vi "GluePattern_Positioning(SubVI)_old.vi"(4 "Duration of glue \ndispensing [s]":dbl=1.5, 5 "File to be processed- Dots":path=path "C:/Users/Aerotech/Documents/BNL_ThermomechanicalStave/1_ModulePlacement/1_GluePatterning/LabVIEW_gluepattern_arraytest.csv", 6 "Type of Pattern":u16(ring) items=["Dots", "Lines"], 7 "Go to \ncoordinates":T5={"X [mm]"=10.0, "Y [mm]"=-17.0, "Z [mm] "=36.0}) -> ()   [LabVIEW 2016]
uses:
  C:/Users/Aerotech/Documents/BNL_ThermomechanicalStave/AerotechLibraries/Bin/Aerotech.A3200.dll
  AerotechLibraries/Bin/Aerotech.A3200.dll
  <vilib>/LabVIEW Interface for Arduino/Type Defs/Arduino Resource.ctl
  <vilib>/LabVIEW Interface for Arduino/Type Defs/Board Type.ctl
  <vilib>/LabVIEW Interface for Arduino/Type Defs/Pin Mode.ctl
  <vilib>/Utility/file.llb/Read Delimited Spreadsheet (DBL).vi
  <vilib>/LabVIEW Interface for Arduino/LabVIEW Interface for Arduino.lvlib
panel:
  out "error out":errorcluster
  out "DX [mm]":dbl
  out "DY [mm]":dbl
  out "Arduino Resource":T1={"VISA resource"="COM3", "Board Type"=enum."Uno", "Connection Type"=enum."USB / Serial", "Bytes Per Packet (15)"=15}
  in  "Digital I/O Pin":u8=7
  in  "Final Z":dbl=41.0
  out "Final Position":T3={"Final X"=10.000061631047261, "Final Y"=-16.999877872052817, "Final Z"=35.999801000000005}
  out "Column":i32
  out "Row":i32
  in  "Home?":bool
  out "XYZ Stage Control":refnum<k24>
  in  "Axis Speeds":T4={"vX [mm]"=40.0, "vY [mm]"=40.0, "vZ [mm] "=40.0}
  in  "Module width [mm]":dbl
  in  "Module length [mm]":dbl
  out "INPUT : Dot":bool[][](array[boolean])=[[TRUE]]
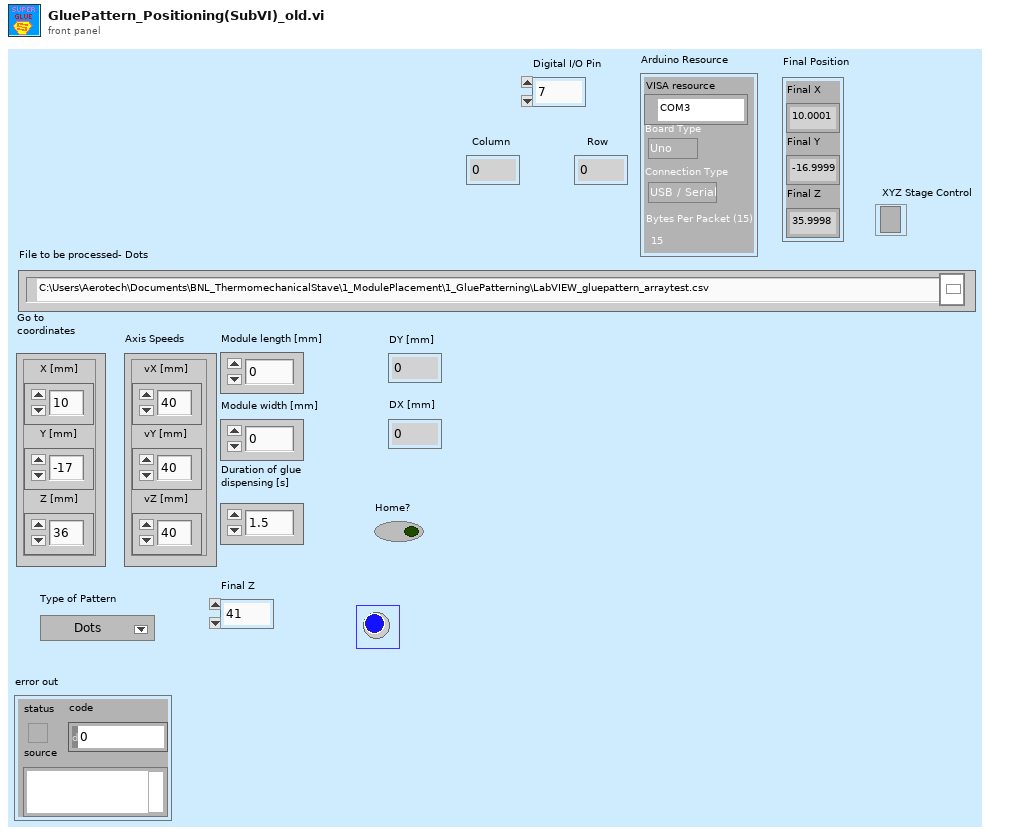
[diagram p1: front panel]
types:
  T1 = typedef "LabVIEW Interface for Arduino.lvlib/Arduino Resource.ctl" = cluster{"VISA resource":refnum<visa-resource-name>, "Board Type":T2, "Connection Type":enum8{"USB / Serial"}, "Bytes Per Packet (15)":u8}
  T2 = typedef "LabVIEW Interface for Arduino.lvlib/Board Type.ctl" = enum16{"Uno", "Dimuelanove w/Atmega 328", "Mega 2560"}
  T3 = cluster{"Final X":dbl, "Final Y":dbl, "Final Z":dbl}
  T4 = cluster{"vX [mm]":dbl, "vY [mm]":dbl, "vZ [mm] ":dbl}
  T5 = cluster{"X [mm]":dbl, "Y [mm]":dbl, "Z [mm] ":dbl}
  T6 = typedef "LabVIEW Interface for Arduino.lvlib/Pin Mode.ctl" = enum8{"Input", "Output"}
  T7 = cluster{"X [mm]":dbl, "Y [mm]":dbl, "Z [mm]":dbl}
  T8 = cluster{"X Position Feedback":dbl, "Y Position Feedback":dbl, "Z Position Feedback":dbl}
  T9 = cluster{"Final X":dbl, "Final Y":dbl, "Z [mm] ":dbl}
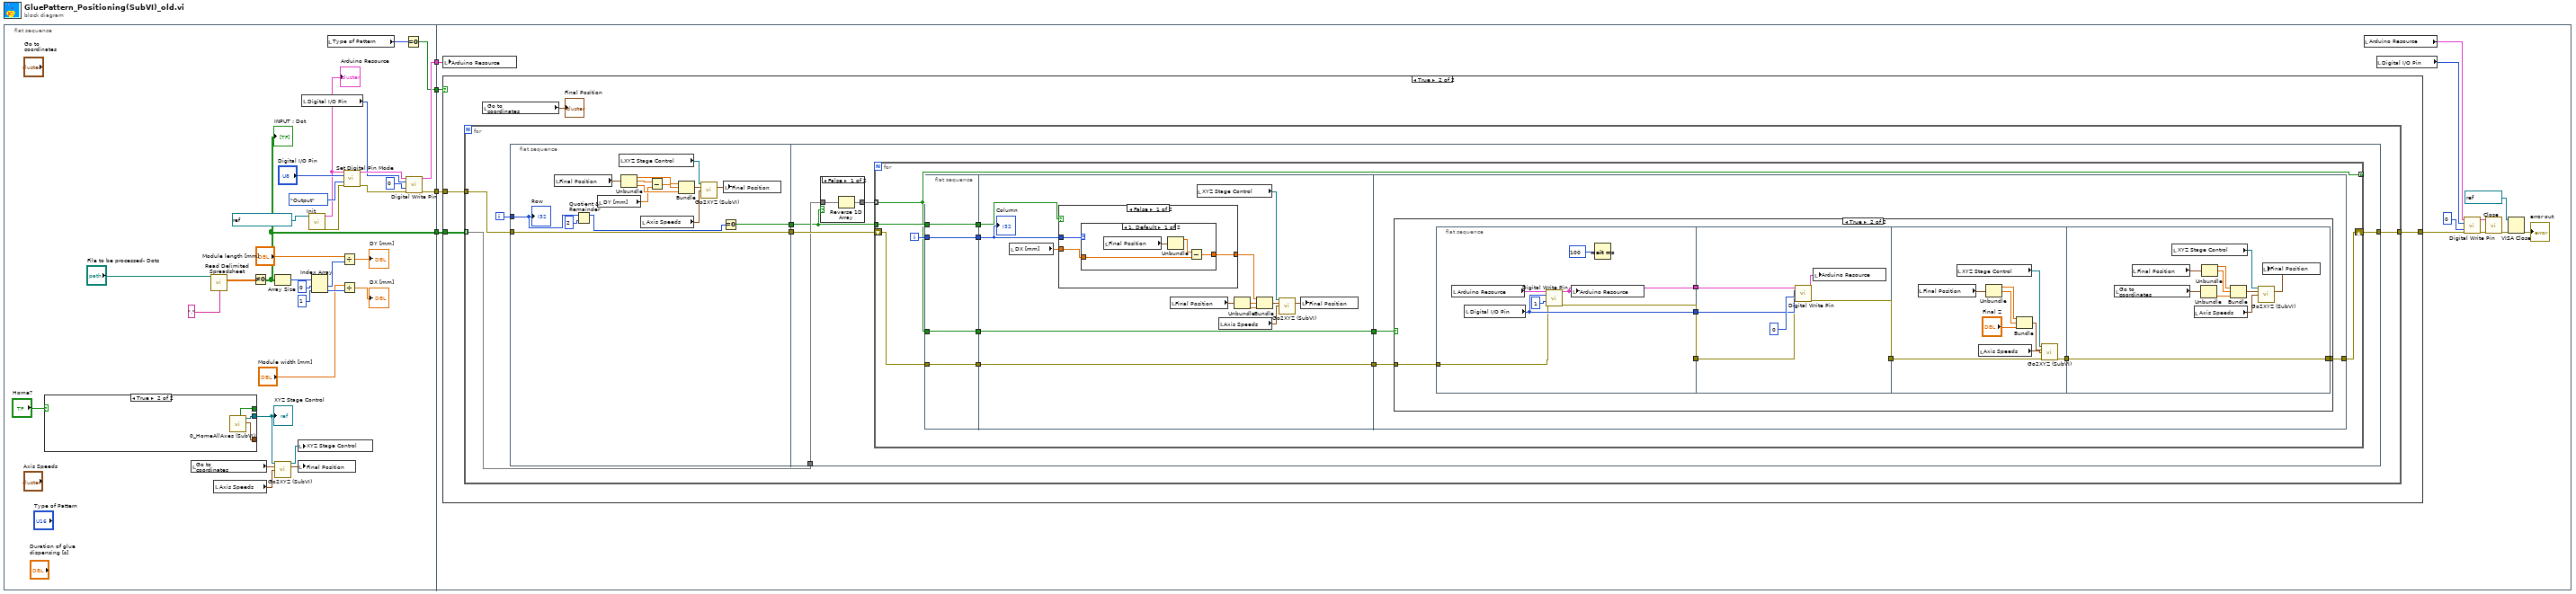
[diagram p0: block diagram]
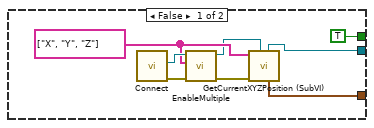
[diagram p2: hidden frame]
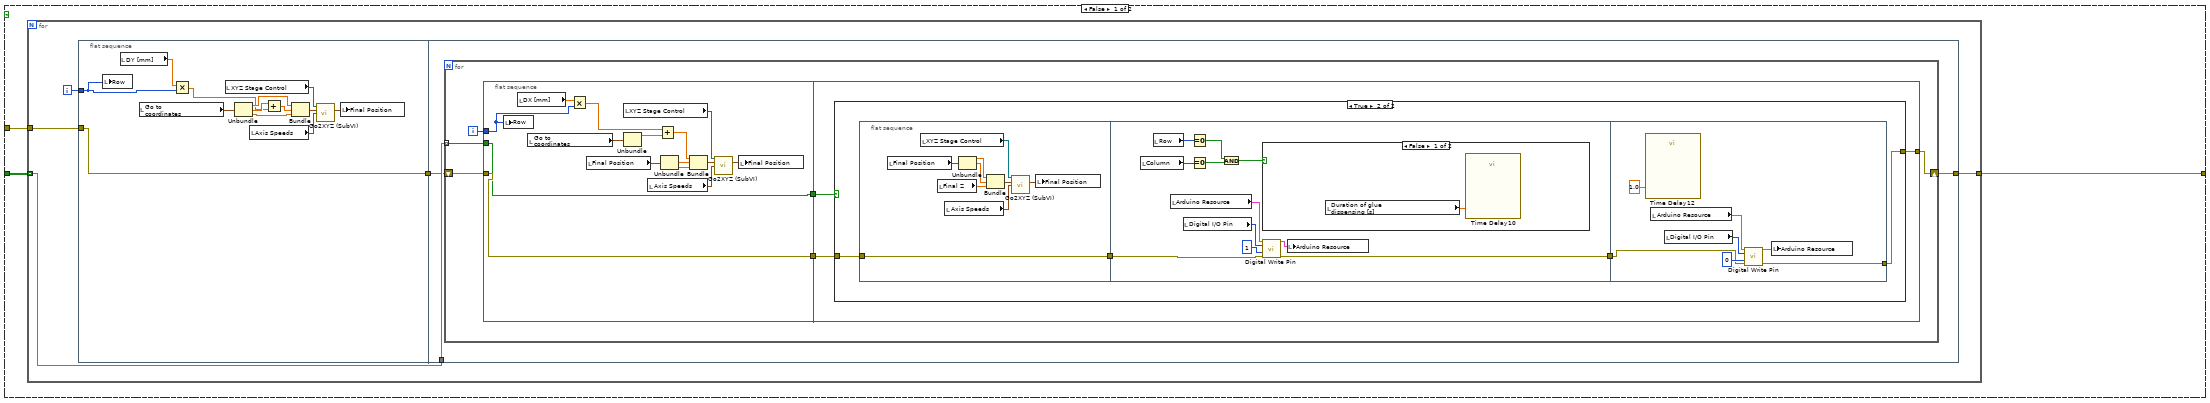
[diagram p3: hidden frame]
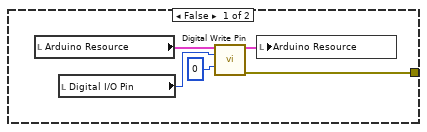
[diagram p4: hidden frame]
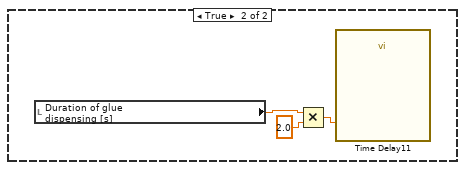
[diagram p5: hidden frame]
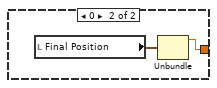
[diagram p7: hidden frame]
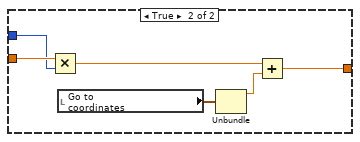
[diagram p8: hidden frame]
diagram:
  n1 = flat-sequence {
    tunnel: [w36] -> w4
    tunnel: [w10] -> w3
    tunnel: [w5] -> w2
    tunnel: [w7] -> w1
    tunnel: w4 -> [w60]
    tunnel: w3 -> [w58]
    tunnel: w2 -> [w59]
    tunnel: w1 -> [w57]
    frame #0 {
      n2 = case shown="True" "Home?" {
        tunnel: [w37 w47] -> _
        tunnel: [TRUE ("completed") w46] -> _
        tunnel: [w39 w45] -> w23
        frame False {
          w41 = string[] ["X", "Y", "Z"] ("Axes Names")
          n3 = call "Connect.vi"() -> ("error out"=w43:errorcluster, "controller"=w42:refnum<k24>)  [unwired: 10 in]
          n4 = call "EnableMultiple.vi"("error in (no error)"=w43, "axis names"=w41, "controller in"=w42) -> ("error out"=w44:errorcluster, "controller out"=w40:refnum<k24>)  [unwired: 7 in]
          n5 = call "GetCurrentXYZPosition (SubVI).vi"(".NET Refnum in - Device"=w40, "error in (no error)"=w44, "Axes Names"=w41) -> ("Current stage position"=w37:T7, ".NET Refnum out  - Device"=w39:refnum<k24>)  [unwired: 3 in, 4 out]
        }
        frame True {
          n6 = call "0_HomeAllAxes (SubVI).vi"() -> ("Homed coordinates"=w47:T8, "controller out"=w45:refnum<k24>, "completed"=w46:bool)  [unwired: 8 in, 1 out]
        }
      }
      "XYZ Stage Control" <- w23
      n7 = local read "Go to \ncoordinates"() -> (w18:T5)
      n8 = call-poly <vilib>:"Read Delimited Spreadsheet.vi"("file path (dialog if empty)"="File to be processed- Dots", "delimiter (\\t)"="," ("delimiter (\\t)")) -> ("all rows"=w34:dbl[][])  [unwired: 8 in, 5 out]
      n9 = local read "Axis Speeds"() -> (w20:T4)
      n10 = Not Equal To 0?(x=w34) -> (x != 0?=w5:bool[][])
      "INPUT : Dot" <- w5
      n11 = Array Size(array=w5) -> (size(s)=w33:i32[])
      n12 = call "Go2XYZ (SubVI).vi"(".NET Refnum in"=w23, "Go to Coordinates"=w18, "Axis Speeds"=w20) -> (".NET Refnum out"=w19:refnum<k24>, "Final Position"=w21:T3)  [unwired: 8 in, 3 out]
      n13 = local write "XYZ Stage Control"(w19) -> ()
      n14 = local write "Final Position"(w21) -> ()
      n15 = local read "Digital I/O Pin"() -> (w9:u8)
      n16 = call <vilib>:"Init.vi"("VISA resource"=refnum<visa-resource-name> "COM3") -> ("Arduino Resource"=w6:T1, "error out"=w11:errorcluster)  [unwired: 17 in]
      "Arduino Resource" <- w6
      n17 = Index Array(array=w33, index #1=0 ("index"), index #2=1 ("index")) -> (element #1=w29:i32, element #2=w28:i32)
      n18 = local read "Type of Pattern"() -> (w8:u16)
      n19 = Divide(x="Module length [mm]", y=w29) -> (x/y=→"DY [mm]":dbl)
      n20 = Divide(x="Module width [mm]", y=w28) -> (x/y=→"DX [mm]":dbl)
      n21 = call <vilib>:"Set Digital Pin Mode.vi"("Arduino Resource"=w6, "Digital I/O Pin"="Digital I/O Pin", "Pin Mode (Input)"=Pin_Mode."Output", "error in"=w11) -> ("Arduino Resource"=w14:T1, "error out"=w15:errorcluster)  [unwired: 10 in]
      n22 = Equal To 0?(x=w8) -> (x = 0?=w7:bool)
      n23 = call <vilib>:"Digital Write Pin.vi"("Arduino Resource"=w14, "Digital I/O Pin (0)"=w9, "Value (0)"=u8 0, "error in"=w15) -> ("Arduino Resource"=w10:T1, "error out"=w36:errorcluster)  [unwired: 10 in]
    }
    frame #1 {
      n24 = local write "Arduino Resource"(w58) -> ()
      n25 = case shown="True" w57 {
        tunnel: w59 -> [w61 w152]
        tunnel: [w62 w151] -> w50
        tunnel: w60 -> [w63 w150]
        frame False {
          n26 = for {
            tunnel: w61 -> [w64] mode=indexing
            tunnel: [w67] -> w62
            tunnel: w63 -> [w65]
            i -> [w68]
            n27 = flat-sequence {
              tunnel: w68 -> [w70]
              tunnel: [w72] -> w66
              tunnel: w65 -> [w72]
              tunnel: w64 -> [w84]
              tunnel: [w83] -> w67
              tunnel: w66 -> [w82]
              frame #0 {
                n28 = local write "Row"(w70) -> ()
                n29 = local read "DY [mm]"() -> (w69:dbl)
                n30 = local read "Go to \ncoordinates"() -> (w78:T5)
                n31 = Multiply(x=w69, y=w70) -> (x*y=w74:dbl)
                n32 = local read "XYZ Stage Control"() -> (w80:refnum<k24>)
                n33 = Unbundle(w78) -> ("X [mm]"=w77:dbl, "Y [mm]"=w75:dbl, "Z [mm]"=w76:dbl)
                n34 = local read "Axis Speeds"() -> (w81:T4)
                n35 = Add(x=w75, y=w74) -> (x+y=w73:dbl)
                n36 = Bundle("X [mm]"=w77, w73, "Z [mm]"=w76) -> (w79:cluster{"X [mm]":dbl, dbl, "Z [mm] ":dbl})  [unwired: 1 in]
                n37 = call "Go2XYZ (SubVI).vi"(".NET Refnum in"=w80, "Go to Coordinates"=w79, "Axis Speeds"=w81) -> ("Final Position"=w71:T3)  [unwired: 8 in, 4 out]
                n38 = local write "Final Position"(w71) -> ()
              }
              frame #1 {
                n39 = for {
                  shift-right: [w85] -> w83
                  shift-left: w82 -> [w89]
                  tunnel: w84 -> [w86] mode=indexing
                  i -> [w90]
                  n40 = flat-sequence {
                    tunnel: w90 -> [w93]
                    tunnel: w89 -> [w103]
                    tunnel: [w103] -> w88
                    tunnel: [w102] -> w87
                    tunnel: w86 -> [w102]
                    tunnel: w88 -> [w108]
                    tunnel: w87 -> [w106]
                    tunnel: [w107] -> w85
                    frame #0 {
                      n41 = local write "Row"(w93) -> ()
                      n42 = local read "DX [mm]"() -> (w91:dbl)
                      n43 = local read "Go to \ncoordinates"() -> (w97:T5)
                      n44 = Multiply(x=w91, y=w93) -> (x*y=w96:dbl)
                      n45 = local read "Final Position"() -> (w92:T3)
                      n46 = local read "XYZ Stage Control"() -> (w104:refnum<k24>)
                      n47 = Unbundle(w97) -> ("X [mm]"=w95:dbl)  [unwired: 2 out]
                      n48 = local read "Axis Speeds"() -> (w105:T4)
                      n49 = Add(x=w96, y=w95) -> (x+y=w94:dbl)
                      n50 = Unbundle(w92) -> ("Final Y"=w101:dbl, "Final Z"=w98:dbl)  [unwired: 1 out]
                      n51 = Bundle(w94, "Final Y"=w101, "Final Z"=w98) -> (w99:cluster{dbl, "Final Y":dbl, "Final Z":dbl})  [unwired: 1 in]
                      n52 = call "Go2XYZ (SubVI).vi"(".NET Refnum in"=w104, "Go to Coordinates"=w99, "Axis Speeds"=w105) -> ("Final Position"=w100:T3)  [unwired: 8 in, 4 out]
                      n53 = local write "Final Position"(w100) -> ()
                    }
                    frame #1 {
                      n54 = case shown="True" w106 {
                        tunnel: [w112 w115] -> w107
                        tunnel: w108 -> [_ w116]
                        frame False {
                          n55 = local read "Arduino Resource"() -> (w111:T1)
                          n56 = local read "Digital I/O Pin"() -> (w110:u8)
                          n57 = call <vilib>:"Digital Write Pin.vi"("Arduino Resource"=w111, "Digital I/O Pin (0)"=w110, "Value (0)"=u8 0) -> ("Arduino Resource"=w109:T1, "error out"=w112:errorcluster)  [unwired: 11 in]
                          n58 = local write "Arduino Resource"(w109) -> ()
                        }
                        frame True {
                          n59 = flat-sequence {
                            tunnel: [w124] -> w117
                            tunnel: w116 -> [w124]
                            tunnel: w117 -> [w132]
                            tunnel: [w136] -> w114
                            tunnel: [w142] -> w115
                            tunnel: w114 -> [w143]
                            frame #0 {
                              n60 = local read "Final Position"() -> (w122:T3)
                              n61 = local read "XYZ Stage Control"() -> (w125:refnum<k24>)
                              n62 = local read "Final Z"() -> (w119:dbl)
                              n63 = local read "Axis Speeds"() -> (w126:T4)
                              n64 = Unbundle(w122) -> ("Final X"=w121:dbl, "Final Y"=w120:dbl)  [unwired: 1 out]
                              n65 = Bundle("Final X"=w121, "Final Y"=w120, "Final Z"=w119) -> (w123:T3)  [unwired: 1 in]
                              n66 = call "Go2XYZ (SubVI).vi"(".NET Refnum in"=w125, "Go to Coordinates"=w123, "Axis Speeds"=w126) -> ("Final Position"=w118:T3)  [unwired: 8 in, 4 out]
                              n67 = local write "Final Position"(w118) -> ()
                            }
                            frame #1 {
                              n68 = local read "Column"() -> (w129:i32)
                              n69 = local read "Row"() -> (w131:i32)
                              n70 = local read "Arduino Resource"() -> (w135:T1)
                              n71 = local read "Digital I/O Pin"() -> (w134:u8)
                              n72 = Equal To 0?(x=w131) -> (x = 0?=w130:bool)
                              n73 = Equal To 0?(x=w129) -> (x = 0?=w128:bool)
                              n74 = And(x=w130, y=w128) -> (x .and. y?=w127:bool)
                              n75 = case shown="False" w127 {
                                frame False {
                                n76 = local read "Duration of glue \ndispensing [s]"() -> (w138:dbl)
                                n77 = call "Time Delay10"("Delay Time (s)"=w138) -> ()  [unwired: 10 in, 1 out]
                                }
                                frame True {
                                n78 = local read "Duration of glue \ndispensing [s]"() -> (w140:dbl)
                                n79 = Multiply(x=w140, y=2.0) -> (x*y=w139:dbl)
                                n80 = call "Time Delay11"("Delay Time (s)"=w139) -> ()  [unwired: 10 in, 1 out]
                                }
                              }
                              n81 = call <vilib>:"Digital Write Pin.vi"("Arduino Resource"=w135, "Digital I/O Pin (0)"=w134, "Value (0)"=u8 1, "error in"=w132) -> ("Arduino Resource"=w133:T1, "error out"=w136:errorcluster)  [unwired: 10 in]
                              n82 = local write "Arduino Resource"(w133) -> ()
                            }
                            frame #2 {
                              n83 = call "Time Delay12"("Delay Time (s)"=1.0) -> ()  [unwired: 10 in, 1 out]
                              n84 = local read "Arduino Resource"() -> (w144:T1)
                              n85 = local read "Digital I/O Pin"() -> (w145:u8)
                              n86 = call <vilib>:"Digital Write Pin.vi"("Arduino Resource"=w144, "Digital I/O Pin (0)"=w145, "Value (0)"=u8 0, "error in"=w143) -> ("Arduino Resource"=w147:T1, "error out"=w142:errorcluster)  [unwired: 10 in]
                              n87 = local write "Arduino Resource"(w147) -> ()
                            }
                          }
                        }
                      }
                    }
                  }
                }
              }
            }
          }
        }
        frame True {
          n88 = for {
            tunnel: w152 -> [w153] mode=indexing
            tunnel: [w157] -> w151
            tunnel: w150 -> [w155]
            i -> [w158]
            n89 = flat-sequence {
              tunnel: w158 -> [w162]
              tunnel: [w173] -> w156
              tunnel: w155 -> [w173]
              tunnel: [w159] -> w154
              tunnel: w153 -> [w176]
              tunnel: [w178] -> w157
              tunnel: w156 -> [w177]
              tunnel: w154 -> [w174]
              frame #0 {
                n90 = local read "Final Position"() -> (w167:T3)
                n91 = Quotient & Remainder(x=w162, y=2) -> (x-y*floor(x/y)=w160:i32)  [unwired: 1 out]
                n92 = local read "DY [mm]"() -> (w163:dbl)
                n93 = local read "XYZ Stage Control"() -> (w165:refnum<k24>)
                n94 = Unbundle(w167) -> ("Final X"=w168:dbl, "Final Y"=w170:dbl, "Final Z"=w169:dbl)
                n95 = local read "Axis Speeds"() -> (w172:T4)
                n96 = Subtract(x=w170, y=w163) -> (x-y=w171:dbl)
                n97 = Bundle("Final X"=w168, w171, "Final Z"=w169) -> (w166:cluster{"Final X":dbl, dbl, "Final Z":dbl})  [unwired: 1 in]
                n98 = call "Go2XYZ (SubVI).vi"(".NET Refnum in"=w165, "Go to Coordinates"=w166, "Axis Speeds"=w172) -> ("Final Position"=w164:T3)  [unwired: 8 in, 4 out]
                n99 = Equal To 0?(x=w160) -> (x = 0?=w159:bool)
                n100 = local write "Final Position"(w164) -> ()
                "Row" <- w162
              }
              frame #1 {
                n101 = case shown="False" w174 {
                  tunnel: w176 -> [w180 w181]
                  tunnel: [w179 w181] -> w175
                  frame False {
                    n102 = Reverse 1D Array(array=w180) -> (reversed array=w179:bool[])
                  }
                  frame True {
                  }
                }
                n103 = for {
                  shift-right: [w188] -> w178
                  shift-left: w177 -> [w191]
                  tunnel: [w182] -> _ mode=indexing
                  tunnel: w174 -> [w187]
                  tunnel: w175 -> [w182] mode=indexing
                  i -> [w192]
                  n104 = flat-sequence {
                    tunnel: w187 -> [w193]
                    tunnel: w182 -> [w194]
                    tunnel: w191 -> [w195]
                    tunnel: w192 -> [w196]
                    tunnel: [w196] -> w186
                    tunnel: [w195] -> w185
                    tunnel: [w194] -> w184
                    tunnel: [w193] -> w183
                    tunnel: [w205] -> w190
                    tunnel: [w197] -> w189
                    tunnel: w186 -> [w206]
                    tunnel: w185 -> [w205]
                    tunnel: w184 -> [w197]
                    tunnel: w183 -> [w198]
                    tunnel: w190 -> [w227]
                    tunnel: w189 -> [w225]
                    tunnel: [w226] -> w188
                    frame #0 {
                    }
                    frame #1 {
                      n105 = local read "DX [mm]"() -> (w207:dbl)
                      n106 = case shown="False" w198 {
                        tunnel: w207 -> [w211 w224]
                        tunnel: w206 -> [w210 w219]
                        tunnel: [w212 w220] -> w199
                        frame False {
                          n107 = case shown="1, Default" w210 {
                            tunnel: [w216 w217] -> w212
                            tunnel: w211 -> [w215 _]
                            frame 1, Default {
                              n108 = local read "Final Position"() -> (w214:T3)
                              n109 = Unbundle(w214) -> ("Final X"=w213:dbl)  [unwired: 2 out]
                              n110 = Subtract(x=w213, y=w215) -> (x-y=w216:dbl)
                            }
                            frame 0 {
                              n111 = local read "Final Position"() -> (w218:T3)
                              n112 = Unbundle(w218) -> ("Final X"=w217:dbl)  [unwired: 2 out]
                            }
                          }
                        }
                        frame True {
                          n113 = Multiply(x=w224, y=w219) -> (x*y=w222:dbl)
                          n114 = local read "Go to \ncoordinates"() -> (w223:T5)
                          n115 = Unbundle(w223) -> ("X [mm]"=w221:dbl)  [unwired: 2 out]
                          n116 = Add(x=w222, y=w221) -> (x+y=w220:dbl)
                        }
                      }
                      n117 = local read "Final Position"() -> (w204:T3)
                      n118 = local read "XYZ Stage Control"() -> (w208:refnum<k24>)
                      n119 = local read "Axis Speeds"() -> (w209:T4)
                      n120 = Unbundle(w204) -> ("Final Y"=w203:dbl, "Final Z"=w200:dbl)  [unwired: 1 out]
                      n121 = Bundle("Final X"=w199, "Final Y"=w203, "Final Z"=w200) -> (w201:T3)  [unwired: 1 in]
                      n122 = call "Go2XYZ (SubVI).vi"(".NET Refnum in"=w208, "Go to Coordinates"=w201, "Axis Speeds"=w209) -> ("Final Position"=w202:T3)  [unwired: 8 in, 4 out]
                      n123 = local write "Final Position"(w202) -> ()
                      "Column" <- w206
                    }
                    frame #2 {
                      n124 = case shown="True" w225 {
                        tunnel: [w228 w234] -> w226
                        tunnel: w227 -> [w228 w235]
                        frame False {
                        }
                        frame True {
                          n125 = flat-sequence {
                            tunnel: w235 -> [w238]
                            tunnel: [w237] -> w232
                            tunnel: [w240] -> w230
                            tunnel: [w239] -> w229
                            tunnel: w232 -> [w244]
                            tunnel: [w243] -> w231
                            tunnel: w230 -> [w248]
                            tunnel: w229 -> [w246]
                            tunnel: [w249] -> w233
                            tunnel: w231 -> [w250]
                            tunnel: [w258] -> w234
                            tunnel: w233 -> [w258]
                            frame #0 {
                              n126 = local read "Arduino Resource"() -> (w241:T1)
                              n127 = local read "Digital I/O Pin"() -> (w239:u8)
                              n128 = call <vilib>:"Digital Write Pin.vi"("Arduino Resource"=w241, "Digital I/O Pin (0)"=w239, "Value (0)"=u8 1, "error in"=w238) -> ("Arduino Resource"=w240:T1, "error out"=w237:errorcluster)  [unwired: 10 in]
                              n129 = local write "Arduino Resource"(w240) -> ()
                              n130 = Wait (ms)(milliseconds to wait=u32 100) -> ()  [unwired: 1 out]
                            }
                            frame #1 {
                              n131 = call <vilib>:"Digital Write Pin.vi"("Arduino Resource"=w248, "Digital I/O Pin (0)"=w246, "Value (0)"=u8 0, "error in"=w244) -> ("Arduino Resource"=w245:T1, "error out"=w243:errorcluster)  [unwired: 10 in]
                              n132 = local write "Arduino Resource"(w245) -> ()
                            }
                            frame #2 {
                              n133 = local read "Final Position"() -> (w253:T3)
                              n134 = local read "XYZ Stage Control"() -> (w255:refnum<k24>)
                              n135 = local read "Axis Speeds"() -> (w256:T4)
                              n136 = Unbundle(w253) -> ("Final X"=w252:dbl, "Final Y"=w251:dbl)  [unwired: 1 out]
                              n137 = Bundle("Final X"=w252, "Final Y"=w251, "Final Z"="Final Z") -> (w254:T3)  [unwired: 1 in]
                              n138 = call "Go2XYZ (SubVI).vi"(".NET Refnum in"=w255, "Go to Coordinates"=w254, "Axis Speeds"=w256, "error in (no error)"=w250) -> ("error out"=w249:errorcluster)  [unwired: 7 in, 4 out]
                            }
                            frame #3 {
                              n139 = local read "Go to \ncoordinates"() -> (w266:T5)
                              n140 = local read "Final Position"() -> (w267:T3)
                              n141 = local read "XYZ Stage Control"() -> (w260:refnum<k24>)
                              n142 = local read "Axis Speeds"() -> (w261:T4)
                              n143 = Unbundle(w266) -> ("Z [mm]"=w263:dbl)  [unwired: 2 out]
                              n144 = Unbundle(w267) -> ("Final X"=w265:dbl, "Final Y"=w264:dbl)  [unwired: 1 out]
                              n145 = Bundle("Final X"=w265, "Final Y"=w264, "Z [mm]"=w263) -> (w262:T9)  [unwired: 1 in]
                              n146 = call "Go2XYZ (SubVI).vi"(".NET Refnum in"=w260, "Go to Coordinates"=w262, "Axis Speeds"=w261) -> ("Final Position"=w259:T3)  [unwired: 8 in, 4 out]
                              n147 = local write "Final Position"(w259) -> ()
                            }
                          }
                        }
                      }
                    }
                  }
                }
              }
            }
          }
          n148 = local read "Go to \ncoordinates"() -> (→"Final Position":T5)
        }
      }
      n149 = local read "Arduino Resource"() -> (w54:T1)
      n150 = local read "Digital I/O Pin"() -> (w55:u8)
      n151 = call <vilib>:"Digital Write Pin.vi"("Arduino Resource"=w54, "Digital I/O Pin (0)"=w55, "Value (0)"=u8 0, "error in"=w50) -> ("Arduino Resource"=w52:T1, "error out"=w51:errorcluster)  [unwired: 10 in]
      n152 = call <vilib>:"Close.vi"("Arduino Resource"=w52, "error in"=w51) -> ("error out"=w49:errorcluster)  [unwired: 13 in]
      n153 = VISA Close(VISA resource name=refnum<visa-resource-name> "COM3", error in (no error)=w49) -> (error out=→"error out":errorcluster)
    }
  }
